vi "CLSUIP_Read New VI.vi"(1 "VIRetooler.lvclass in":refnum<class "VIRetooler.lvclass">) -> (0 "New VI":refnum<vi>)   [LabVIEW 2021, in "MemberVICreation.lvlib" / "VIRetooler.lvclass"]
uses:
  <resource>/Framework/Providers/LVClassLibrary/NewAccessors/VIRetooler/VIRetooler.lvclass
  <resource>/Framework/Providers/LVClassLibrary/NewAccessors/VIRetooler/VIRetooler.lvclass/VIRetooler.ctl
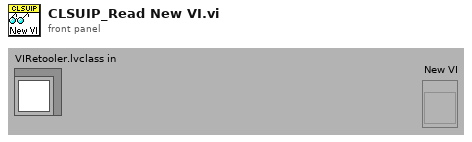
[diagram p1: front panel]
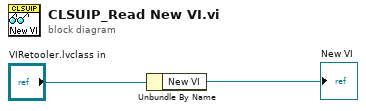
[diagram p0: block diagram]
diagram:
  n1 = Unbundle By Name("VIRetooler.lvclass in") -> ("New VI"=→"New VI":refnum<vi>)
